vi "Log Creation.vi"(8 "error in (no error)":errorcluster, 10 "Log Type":T1, 11 "CIFCorePlugin in":refnum<class "CIFCorePlugin.lvclass">) -> (0 "error out":errorcluster, 3 "CIFCorePlugin out":refnum<class "CIFCorePlugin.lvclass">)   [LabVIEW 2021, in "CIFCorePlugin.lvclass"]
uses:
  CIFCorePlugin.lvclass
  Typedef/Log Type.ctl
  CIFCorePlugin.lvclass/CIFCorePlugin.ctl
  CIFUtilities/CIFLogs/Typedef/Plugin State Commands.ctl
  Accessors/Read Plugin Name.vi
  Accessors/Read gRPC Server Port.vi
  Accessors/Read Version.vi
  CIFUtilities/CIFLogs/CIFLogs.lvlib
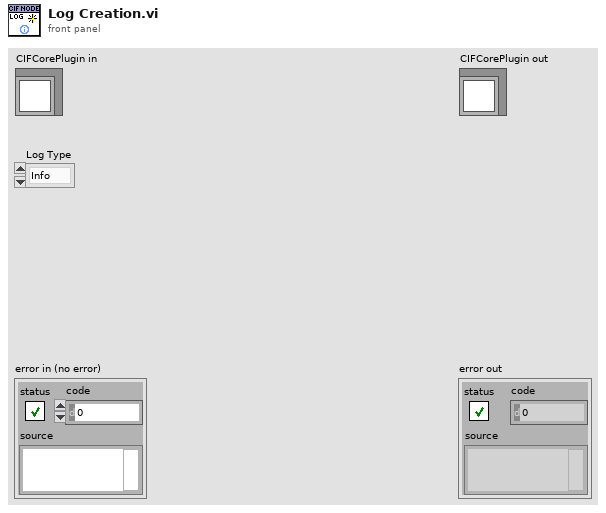
[diagram p1: front panel]
types:
  T1 = typedef "CIFCorePlugin.lvclass/Log Type.ctl" = enum16{"Info", "Config"}
  T2 = typedef "Plugin State Commands.ctl" = enum16{"Create", "Run", "Pause", "Destroy"}
  T3 = typedef "CIFCoreCommon.lvlib/Version.ctl" = cluster{"Major":i32, "Minor":i32, "Fix":i32, "Build":i32}
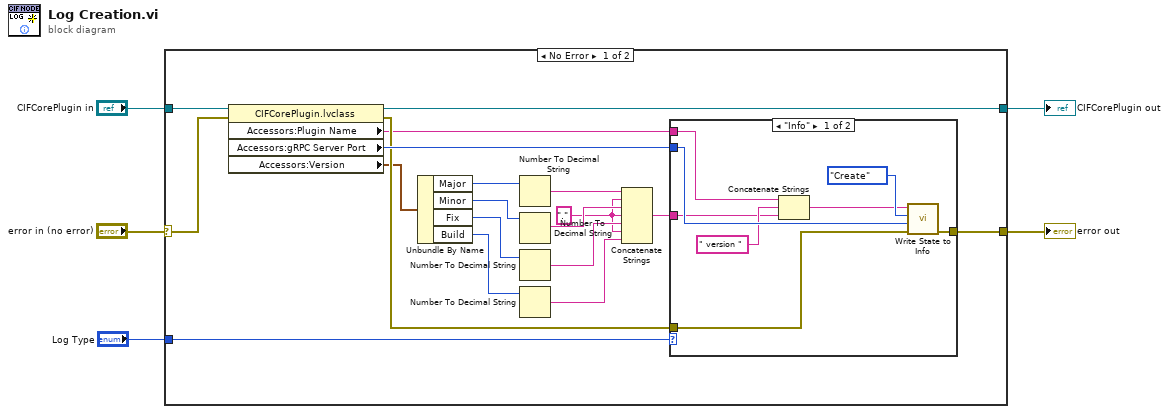
[diagram p0: block diagram]
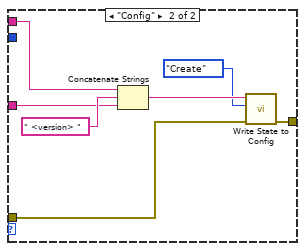
[diagram p2: hidden frame]
diagram:
  n1 = case shown="No Error" "error in (no error)" {
    selector: "error in (no error)" -> [w19 w41]
    tunnel: [w20 w41] -> w4
    tunnel: [w22 w40] -> w2
    tunnel: "CIFCorePlugin in" -> [w24 w40]
    tunnel: "Log Type" -> [w6 _]
    frame No Error {
      w11 = "."
      n2 = property class="CIFCorePlugin.lvclass"(reference=w24, error in=w19) -> (reference out=w22:refnum<class "CIFCorePlugin.lvclass">, error out=w21:errorcluster, "Accessors:Plugin Name"=w8:string, "Accessors:gRPC Server Port"=w23:i32, "Accessors:Version"=w9:T3)
      n3 = Unbundle By Name(w9) -> ("Major"=w18:i32, "Minor"=w17:i32, "Fix"=w13:i32, "Build"=w14:i32)
      n4 = Number To Decimal String(number=w18) -> (decimal integer string=w16:string)  [unwired: 1 in]
      n5 = Number To Decimal String(number=w17) -> (decimal integer string=w15:string)  [unwired: 1 in]
      n6 = Number To Decimal String(number=w13) -> (decimal integer string=w12:string)  [unwired: 1 in]
      n7 = Number To Decimal String(number=w14) -> (decimal integer string=w10:string)  [unwired: 1 in]
      n8 = Concatenate Strings(w16, w11, w15, w11, w12, w11, w10) -> (w7:string)
      n9 = case shown="\"Info\"" w6 {
        tunnel: w23 -> [w32 _]
        tunnel: w21 -> [w30 w36]
        tunnel: [w29 w33] -> w20
        tunnel: w8 -> [w28 w39]
        tunnel: w7 -> [w26 w37]
        frame "Info" {
          n10 = Concatenate Strings(w28, " version " ("string"), w26) -> (w25:string)
          n11 = call "Write State to Info.vi"("error in (no error)"=w30, "gRPC Port"=w32, "Command"=Plugin_State_Commands."Create", "Plugin Name"=w25) -> ("error out"=w29:errorcluster)  [unwired: 7 in]
        }
        frame "Config" {
          n12 = Concatenate Strings(w39, " <version> " ("string"), w37) -> (w35:string)
          n13 = call "Write State to Config.vi"("error in (no error)"=w36, "Command"=Plugin_State_Commands."Create", "Plugin Name"=w35) -> ("error out"=w33:errorcluster)  [unwired: 8 in]
        }
      }
    }
    frame Error {
    }
  }
  "error out" <- w4
  "CIFCorePlugin out" <- w2
